vi "Get All Pin Names - Cached.vi"(0 "TSM Context in":T1, 1 "Reload Cache?":bool caption="Reload Cache? (F)", 11 "error in":errorcluster) -> (4 "Pin Types":T2[](array[typedef]), 6 "Pin Names":tag[](array[tag]), 15 "error out":errorcluster)   [LabVIEW 2019]
uses:
  TSM Pin Type Identifier.ctl
  <vilib>/NI_TestStand_SemiconductorModule/NI_TestStand_Semiconductor_Module.lvlibp/PinMap/General/SemiconductorModuleContext.ctl
  <vilib>/NI_TestStand_SemiconductorModule/NI_TestStand_Semiconductor_Module.lvlibp
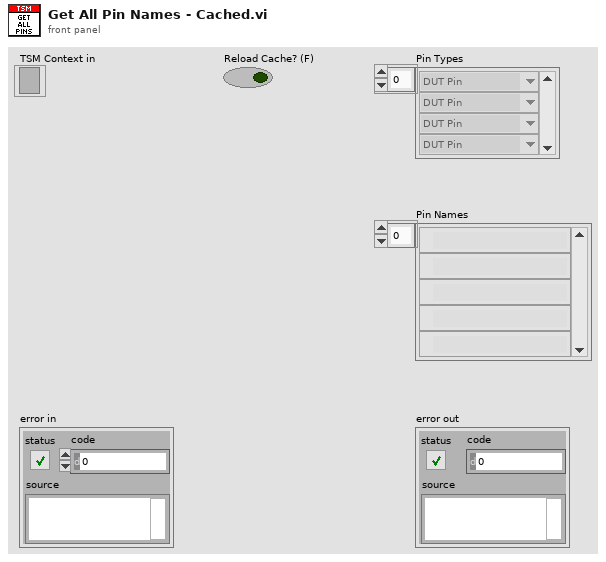
[diagram p1: front panel]
types:
  T1 = typedef "NI_TestStand_Semiconductor_Module.lvlibp/SemiconductorModuleContext.ctl" = refnum<k7>
  T2 = typedef "TSM Pin Type Identifier.ctl" = enum8{"DUT Pin", "System Pin", "Pin Group", "Not Determined"}
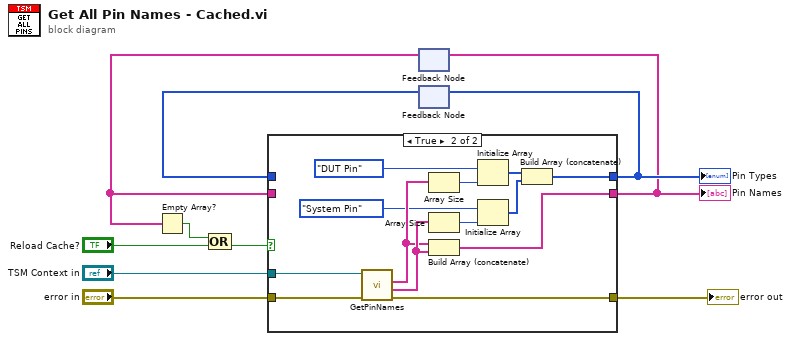
[diagram p0: block diagram]
diagram:
  n1 = feedback #1() -> (w2:tag[])  [unwired: 1 in]
  n2 = Empty Array?(array=w2) -> (empty?=w1:bool)
  n3 = Compound Arithmetic op=OR(w1, "Reload Cache?") -> (w4:bool)
  n4 = feedback #2() -> (w3:T2[])  [unwired: 1 in]
  n5 = case shown="True" w4 {
    tunnel: [w11 w18] -> w5
    tunnel: [w12 w17] -> w6
    tunnel: "TSM Context in" -> [_ w16]
    tunnel: [w13 w15] -> w9
    tunnel: "error in" -> [w13 w14]
    tunnel: w3 -> [w12 _]
    tunnel: w2 -> [w11 _]
    frame False {
    }
    frame True {
      n6 = call <vilib>:"GetPinNames.vi"("error in (no error)"=w14, "Semiconductor Module Context"=w16) -> ("error out"=w15:errorcluster, "System Pins"=w22:tag[], "DUT Pins"=w21:tag[])  [unwired: 6 in, 1 out]
      n7 = Array Size(array=w21) -> (size(s)=w24:i32)
      n8 = Array Size(array=w22) -> (size(s)=w23:i32)
      n9 = Build Array (concatenate)(w21, w22) -> (w18:tag[])
      n10 = Initialize Array(TSM_Pin_Type_Identifier."DUT Pin" ("Enum"), w24) -> (w25:T2[])
      n11 = Initialize Array(TSM_Pin_Type_Identifier."System Pin" ("Enum"), w23) -> (w26:T2[])
      n12 = Build Array (concatenate)(w25, w26) -> (w17:T2[])
    }
  }
  "Pin Names" <- w5
  "Pin Types" <- w6
  "error out" <- w9
  n13 = feedback-in #1(w5) -> ()
  n14 = feedback-in #2(w6) -> ()
